vi "DisplayBottomControl_DP_Ver5.0.vi"(0 "Control Ring Array":refnum<vi>[](array[refnum]), 1 "XYGraph Refnum":refnum<vi>, 3 "Scale Arr Refnum":refnum<vi>, 4 "Title Name Array":string[](array[string])) -> (6 "Y Ref. Output":refnum<vi>[](array[refnum]), 7 "dup Scale Arr Refnum":refnum<vi>, 8 "XY WFGraph Ref.":refnum<vi>)   [LabVIEW 2012]
doc: "This is a subVI to control the disablement and the display items on the X, Y control Ring. \"Control Ring Ref.\" Cluster have to follow the order showed as follow:\n0: X axis control ring\n1: y1 control ring\n2: y2 control ring \n ........\n\"Title Name array\" is the item name which will be showed on the control ring\nIt's # of elements also controls how many contro ring are going to enable."
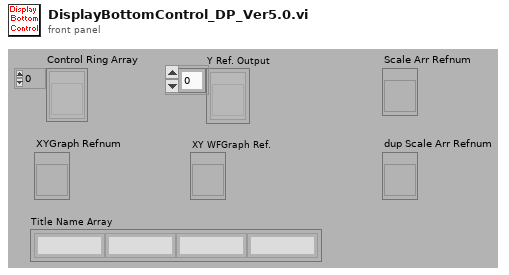
[diagram p1: front panel]
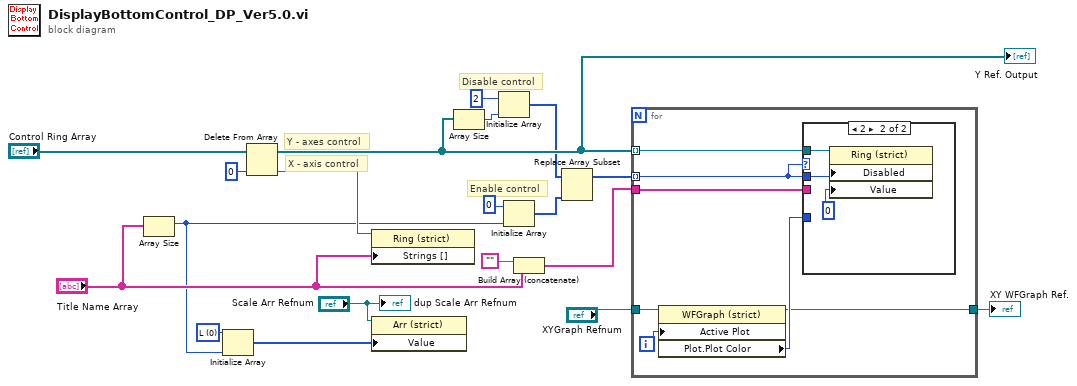
[diagram p0: block diagram]
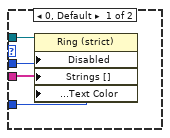
[diagram p2: hidden frame]
diagram:
  w4 = u16 0 items=["L", "R"] ("Y-axes slector 2")
  # "X - axis control"
  # "Y - axes control"
  # "Disable control"
  # "Enable control"
  n1 = Array Size(array="Title Name Array") -> (size(s)=w3:i32)
  n2 = Initialize Array(w4, w3) -> (w1:u16[])
  n3 = Delete From Array(array="Control Ring Array", index=0) -> (deleted portion=w19:refnum<vi>, array with subset deleted=w18:refnum<vi>[])  [unwired: 1 in]
  "Y Ref. Output" <- w18
  n4 = property class="Ring (strict)"(reference=w19, "Strings []"="Title Name Array") -> ()  [unwired: 1 in, 2 out]
  n5 = property class="Arr (strict)"(reference="Scale Arr Refnum", "Value"=w1) -> ()  [unwired: 1 in, 2 out]
  n6 = Array Size(array=w18) -> (size(s)=w10:i32)
  n7 = Initialize Array(2, w10) -> (w12:i32[])
  n8 = Initialize Array(0, w3) -> (w13:i32[])
  n9 = Build Array (concatenate)("", "Title Name Array") -> (w16:string[])
  n10 = Replace Array Subset(array=w12, new element=w13) -> (w14:i32[])  [unwired: 1 in]
  n11 = for {
    tunnel: w14 -> [w25] mode=indexing
    tunnel: w18 -> [w26] mode=indexing
    tunnel: w16 -> [w24]
    tunnel: "XYGraph Refnum" -> [w23]
    tunnel: [w20] -> w6
    i -> [w22]
    n12 = property class="WFGraph (strict)"(reference=w23, "Active Plot"=w22) -> (reference out=w20:refnum<vi>, "Plot.Plot Color"=w21:u32)  [unwired: 1 in, 1 out]
    n13 = case shown="2" w25 {
      tunnel: w26 -> [w30 w33]
      tunnel: w25 -> [w29 w32]
      tunnel: w24 -> [w28 _]
      tunnel: w21 -> [w27 _]
      frame 0, Default {
        n14 = property class="Ring (strict)"(reference=w30, "Disabled"=w29, "Strings []"=w28, "Named Numeric Colors:Text Color"=w27) -> ()  [unwired: 1 in, 2 out]
      }
      frame 2 {
        n15 = property class="Ring (strict)"(reference=w33, "Disabled"=w32, "Value"=u8 0) -> ()  [unwired: 1 in, 2 out]
      }
    }
  }
  "XY WFGraph Ref." <- w6
  "dup Scale Arr Refnum" <- "Scale Arr Refnum"
